vi "Single_Measurement_Main_v2.vi"(7 "Config files paths":T1={"ZI config file (.ini)"="Config_Ver_2\\Zurich_params.ini", "Keithley config file (.ini)"="Config_Ver_2\\Keithley_params.ini", "DAQ config file (.ini)"="Config_Ver_2\\pulse_sequence_DAQ.ini"}, 8 "error in":errorcluster, 10 "Timeout [ms]":u64=5000 min=4000, 11 "Resources in":T2={"ZI Handle"={"handleValid"=FALSE, "Conn"=0, "Path Prefix"="", "Handle"=0, "Clockbase(s)"=0.0, "Connected"=FALSE}, "ZI ModHandle"={"handleValid"=FALSE, "Conn"=0, "ModHandle"=0, "moduleID"="", "Path Prefix"=""}, "VISA Keithley"="KEITHLEY"} {"ZI ModHandle"."ModHandle" format="0x%08x"; "ZI ModHandle"."Conn" format="0x%08x"; "ZI Handle"."Handle" format="0x%08x"; "ZI Handle"."Conn" format="0x%08x"}) -> (0 "error out":errorcluster, 2 "progress":dbl(slide) scale=0.0..1.0, 3 "Resources out":T2 {"ZI ModHandle"."ModHandle" format="0x%08x"; "ZI ModHandle"."Conn" format="0x%08x"; "ZI Handle"."Handle" format="0x%08x"; "ZI Handle"."Conn" format="0x%08x"})   [LabVIEW 2021]
uses:
  Resources_v2.ctl
  <instrlib>/Zurich Instruments LabOne/Public/ziTypeHandle.ctl
  <instrlib>/Zurich Instruments LabOne/Public/Modules/ziTypeModHandle.ctl
  Config_File_Paths_v2.ctl
  <instrlib>/Keithley 622x LV 2009/Typedefs/KE622x -- On Off Control.ctl
  <vilib>/Utility/error.llb/Error Cluster From Error Code.vi
  <vilib>/ErrorRing/Error Ring.xnode
  <instrlib>/Zurich Instruments LabOne/Zurich Instruments LabOne.lvlib
  <instrlib>/Keithley 622x LV 2009/Keithley 622x.lvlib
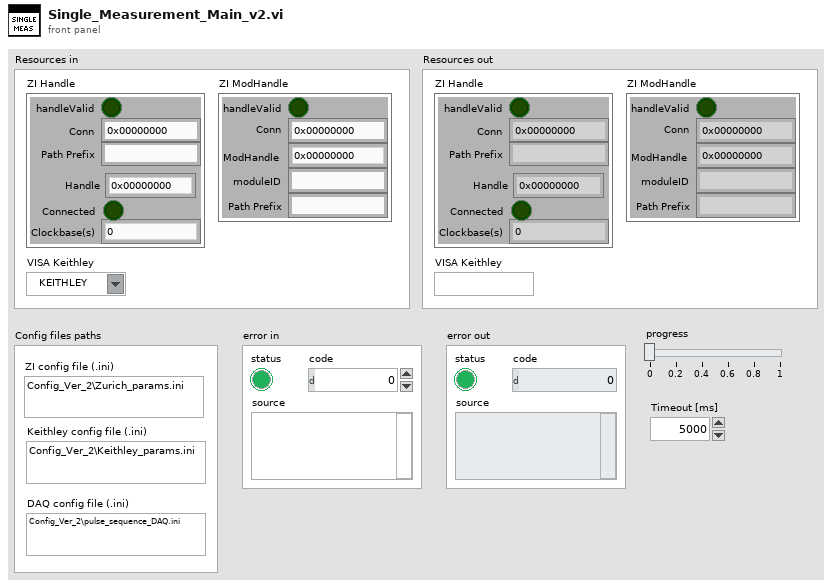
[diagram p1: front panel]
types:
  T1 = typedef "Config_File_Paths_v2.ctl" = cluster{"ZI config file (.ini)":string, "Keithley config file (.ini)":string, "DAQ config file (.ini)":string}
  T2 = typedef "Resources_v2.ctl" = cluster{"ZI Handle":T3, "ZI ModHandle":T4, "VISA Keithley":refnum<visa-resource-name>}
  T3 = typedef "Zurich Instruments LabOne.lvlib/ziTypeHandle.ctl" = cluster{"handleValid":bool, "Conn":u64, "Path Prefix":string, "Handle":u64, "Clockbase(s)":dbl, "Connected":bool}
  T4 = typedef "Zurich Instruments LabOne.lvlib/ziTypeModHandle.ctl" = cluster{"handleValid":bool, "Conn":u64, "ModHandle":u64, "moduleID":string, "Path Prefix":string}
  T5 = typedef "Keithley 622x.lvlib/KE622x -- On Off Control.ctl" = enum16{"Off", "On"}
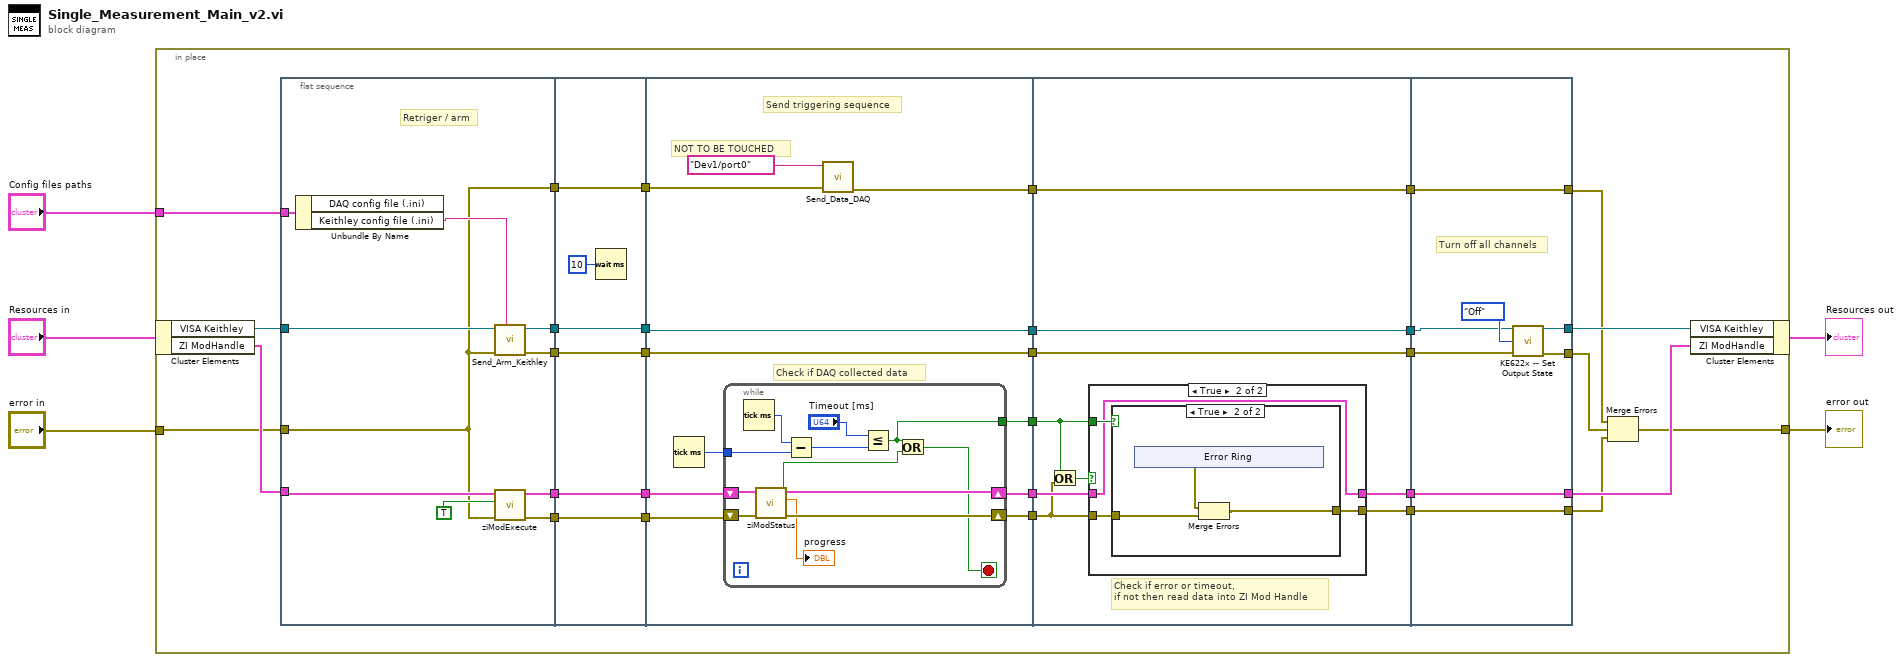
[diagram p0: block diagram]
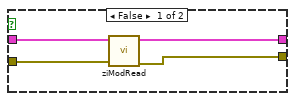
[diagram p2: hidden frame]
diagram:
  n1 = in-place {
    in-place-border: "Config files paths" -> [w34]
    in-place-border: "error in" -> [w33]
    in-place-border: [w6] -> w4
    n2 = in-place-cluster #1("Resources in") -> ("VISA Keithley"=w35:refnum<visa-resource-name>, "ZI ModHandle"=w36:T4)
    n3 = flat-sequence {
      tunnel: w36 -> [w45]
      tunnel: w35 -> [w46]
      tunnel: w34 -> [w43]
      tunnel: w33 -> [w37]
      tunnel: [w37] -> w31
      tunnel: [w41] -> w29
      tunnel: [w40] -> w27
      tunnel: [w39] -> w25
      tunnel: [w38] -> w23
      tunnel: [w51] -> w32
      tunnel: w31 -> [w51]
      tunnel: [w50] -> w30
      tunnel: w29 -> [w50]
      tunnel: [w49] -> w28
      tunnel: w27 -> [w49]
      tunnel: [w48] -> w26
      tunnel: w25 -> [w48]
      tunnel: [w47] -> w24
      tunnel: w23 -> [w47]
      tunnel: w32 -> [w55]
      tunnel: w30 -> [w60]
      tunnel: w28 -> [w59]
      tunnel: w26 -> [w63]
      tunnel: w24 -> [w62]
      tunnel: [w54] -> w22
      tunnel: [w60] -> w21
      tunnel: [w59] -> w20
      tunnel: [w58] -> w19
      tunnel: [w57] -> w18
      tunnel: [w56] -> w17
      tunnel: w22 -> [w84]
      tunnel: w21 -> [w83]
      tunnel: w20 -> [w82]
      tunnel: w19 -> [w80]
      tunnel: w18 -> [w79]
      tunnel: w17 -> [w76]
      tunnel: [w84] -> w16
      tunnel: [w83] -> w15
      tunnel: [w82] -> w14
      tunnel: [w78] -> w13
      tunnel: [w77] -> w12
      tunnel: [w108] -> w9
      tunnel: [w109] -> w10
      tunnel: w16 -> [w102]
      tunnel: w15 -> [w106]
      tunnel: w14 -> [w105]
      tunnel: w13 -> [w109]
      tunnel: w12 -> [w108]
      tunnel: [w104] -> w11
      tunnel: [w102] -> w7
      tunnel: [w103] -> w8
      frame #0 {
        # "Retriger / arm"
        n4 = Unbundle By Name(w43) -> ("Keithley config file (.ini)"=w42:string)  [unwired: 1 out]
        n5 = call "Send_Arm_Keithley.vi"("Filename (.ini)"=w42, "error in"=w37, "Keithley VISA in"=w46) -> ("error out"=w40:errorcluster, "Keithley VISA out"=w41:refnum<visa-resource-name>)  [unwired: 6 in, 1 out]
        n6 = call <instrlib>:"ziModExecute.vi"("Error In"=w37, "Modal (F)"=TRUE, "ziModHandle In"=w45) -> ("Error Out"=w38:errorcluster, "ziModHandle Out"=w39:T4)  [unwired: 6 in]
      }
      frame #1 {
        n7 = Wait (ms)(milliseconds to wait=u32 10) -> ()  [unwired: 1 out]
      }
      frame #2 {
        # "NOT TO BE TOUCHED"
        # "Check if DAQ collected data"
        # "Send triggering sequence"
        n8 = Tick Count (ms)() -> (millisecond timer value=w61:u32)
        n9 = while {
          shift-right: [w74] -> w57
          shift-left: w63 -> [w75]
          shift-right: [w72] -> w56
          shift-left: w62 -> [w73]
          tunnel: w61 -> [w69]
          tunnel: [w64] -> w58
          stop <- w65 stop-if-true
          n10 = Tick Count (ms)() -> (millisecond timer value=w70:u32)
          n11 = call <instrlib>:"ziModStatus.vi"("Error In"=w73, "ModHandle IN"=w75) -> ("Error Out"=w72:errorcluster, "Finished?"=w66:bool, "Progress (unity)"=→"progress":dbl, "ModHandle Out"=w74:T4)  [unwired: 5 in]
          n12 = Subtract(x=w70, y=w69) -> (x-y=w68:u32)
          n13 = Less Or Equal?(x="Timeout [ms]", y=w68) -> (x <= y?=w64:bool)
          n14 = Or(x=w64, y=w66) -> (x .or. y?=w65:bool)
        }
        n15 = call "Send_Data_DAQ.vi"("error in"=w55, "Digital Ports"=tag "Dev1/port0") -> ("error out"=w54:errorcluster)  [unwired: 8 in, 1 out]
      }
      frame #3 {
        # "Check if error or timeout,\nif not then read data into ZI Mod Handle"
        n16 = Or(x=w80, y=w76) -> (x .or. y?=w81:bool)
        n17 = case shown="True" w81 {
          tunnel: w76 -> [w87 w91]
          tunnel: w80 -> [_ w92]
          tunnel: [w86 w90] -> w77
          tunnel: w79 -> [w88 w89]
          tunnel: [w85 w89] -> w78
          frame False {
            n18 = call <instrlib>:"ziModRead.vi"("error in"=w87, "ziModHandle In"=w88) -> ("error out"=w86:errorcluster, "ziModHandle Out"=w85:T4)  [unwired: 8 in]
          }
          frame True {
            n19 = case shown="True" w92 {
              tunnel: w91 -> [w93 w95]
              tunnel: [w93 w94] -> w90
              frame False {
              }
              frame True {
                n20 = xnode "Error Ring"() -> ("error out"=w96:errorcluster)
                n21 = Merge Errors(w96, w95) -> (w94:errorcluster)
              }
            }
          }
        }
      }
      frame #4 {
        # "Turn off all channels"
        n22 = call <instrlib>:"KE622x -- Set Output State.vi"("Resource In"=w106, "Output State"=KE622x_--_On_Off_Control."Off", "error in (no error)"=w105) -> ("Resource Out (dupl)"=w104:refnum<visa-resource-name>, "error out"=w103:errorcluster)  [unwired: 11 in]
      }
    }
    n23 = Merge Errors(w7, w8, w9) -> (w6:errorcluster)
    n24 = in-place-cluster #1("VISA Keithley"=w11, "ZI ModHandle"=w10) -> (→"Resources out":T2)
  }
  "error out" <- w4
